vi "Movement control REVISED.vi"() -> ()   [LabVIEW 2018]
panel:
  out "Speed":T1
  in  "stop":bool
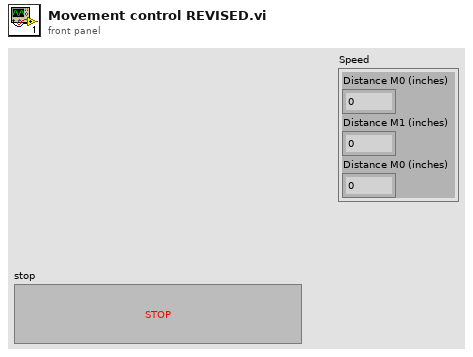
[diagram p1: front panel]
types:
  T1 = cluster{"Distance M0 (inches)":dbl, "Distance M1 (inches)":dbl, "Distance M0 (inches)":dbl}
  T2 = cluster{"Distance M0 ":dbl, "Distance M1 ":dbl, "Distance M2 ":dbl}
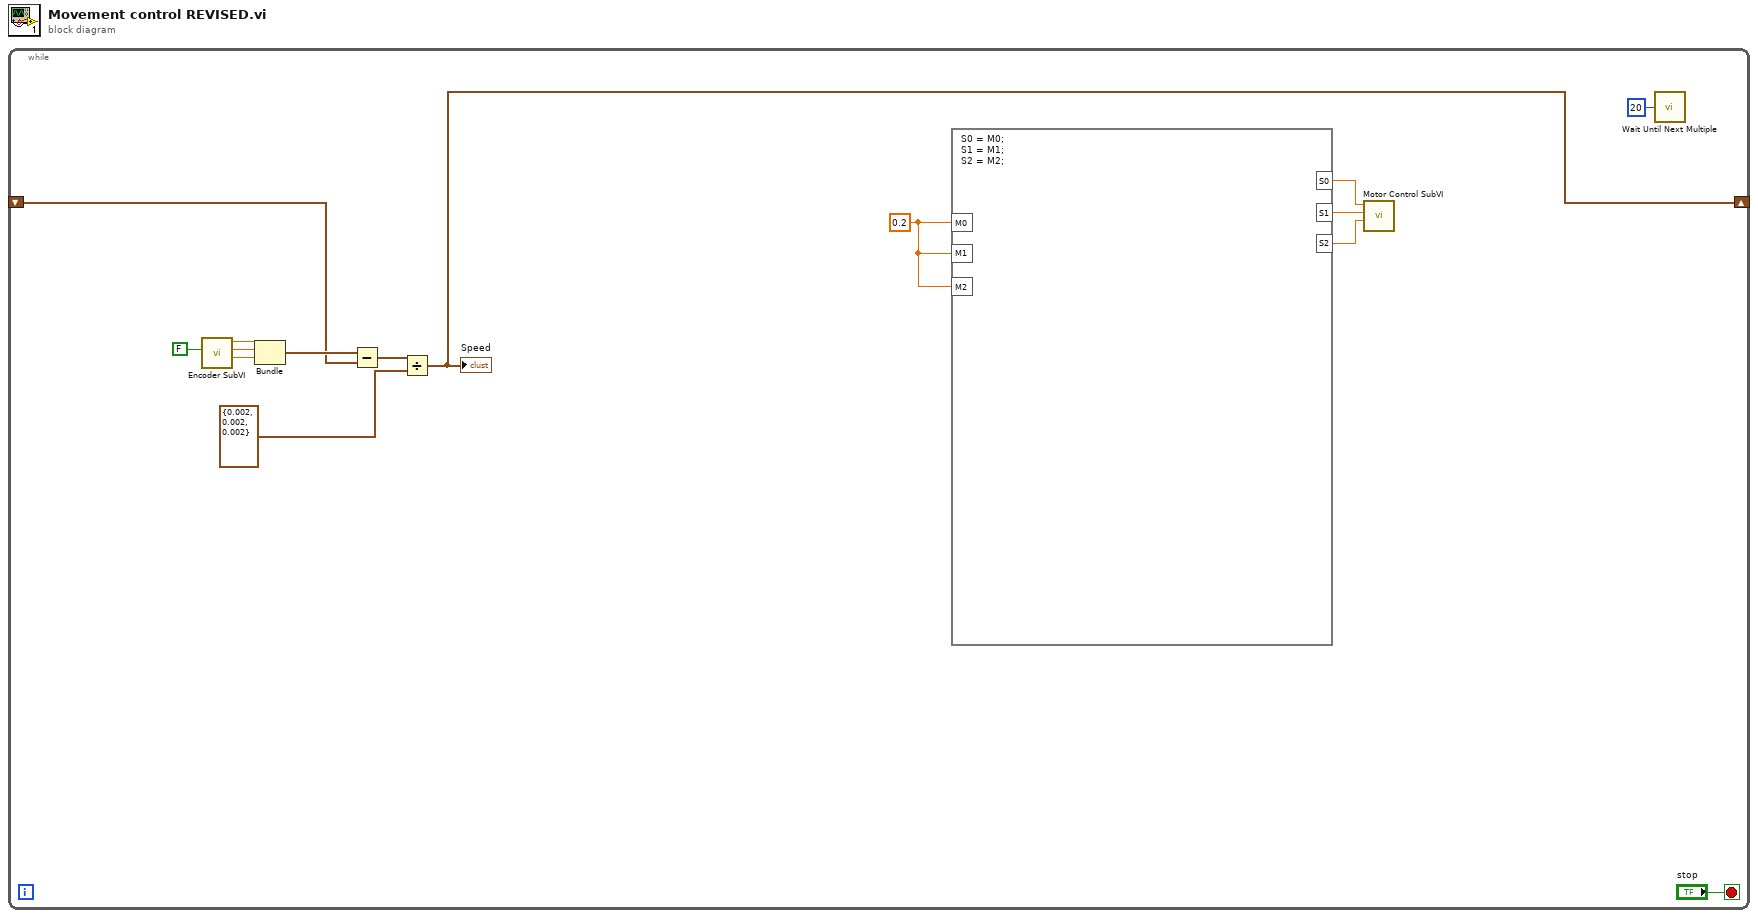
[diagram p0: block diagram]
diagram:
  n1 = while {
    shift-right: [w2] -> _
    shift-left: _ -> [w3]
    stop <- "stop" stop-if-true
    w11 = 0.2 ("input variable")
    n2 = call "Encoder SubVI.vi"("Reset Encoders"=FALSE ("Reset Encoder 0")) -> ("Distance M2"=w5:dbl, "Distance M1"=w6:dbl, "Distance M0"=w7:dbl)  [unwired: 7 in, 1 out]
    n3 = Bundle("Distance M0"=w7, "Distance M1"=w6, "Distance M2"=w5) -> (w4:T2)  [unwired: 1 in]
    n4 = Subtract(x=w4, y=w3) -> (x-y=w13:cluster{dbl, dbl, dbl})
    n5 = Divide(x=w13, y=T1 {"Distance M0 (inches)"=0.002, "Distance M1 (inches)"=0.002, "Distance M0 (inches)"=0.002}) -> (x/y=w2:cluster{dbl, dbl, dbl})
    "Speed" <- w2
    n6 = formula code="S0 = M0;\nS1 = M1;\nS2 = M2;"("M0"=w11, "M1"=w11, "M2"=w11) -> ("S0"=w10:dbl, "S1"=w9:dbl, "S2"=w8:dbl)
    n7 = call "Motor Control SubVI.vi"("Speed M2"=w8, "Speed M1"=w9, "Speed M0"=w10) -> ()  [unwired: 8 in, 1 out]
    n8 = call "Wait Until Next Multiple"("Count(Ticks)"=u32 20) -> ()  [unwired: 1 out]
  }
